vi "ELVIS III v1.0 Unreserve DI Block.vi"(7 "Allow multiple opens?":bool, 8 "error in (no error)":errorcluster, 10 "DI (N Samples) Channel List":T2, 11 "Generic FPGA Reference":T1) -> (0 "error out":errorcluster)   [LabVIEW 2021]
uses:
  <vilib>/myRIO/Common/Instrument Driver Framework/myRIO v1.0/DI Block/typedefs/DI Block Channels List.ctl
  <vilib>/myRIO/Common/Instrument Driver Framework/myRIO v1.0/DI Block/typedefs/DI Block Channels Enum.ctl
  <vilib>/myRIO/Common/Instrument Driver Framework/Utilities/typedefs/Generic FPGA Reference.ctl
  <vilib>/myRIO/Common/Instrument Driver Framework/ELVIS III v1.0/Resource Manager/vis/ELVIS III v1.0 Create Configuration List.vi
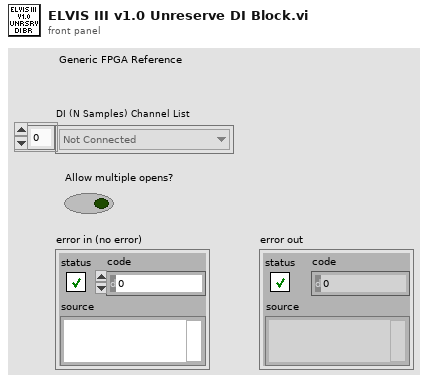
[diagram p1: front panel]
types:
  T1 = typedef "Generic FPGA Reference.ctl" = refnum<k20>
  T2 = typedef "DI Block Channels List.ctl" = T3[]
  T3 = typedef "DI Block Channels Enum.ctl" = enum16{"Not Connected", "A/DI0 (N Samples)", "A/DI1 (N Samples)", "A/DI2 (N Samples)", "A/DI3 (N Samples)", "A/DI4 (N Samples)", "A/DI5 (N Samples)", "A/DI6 (N Samples)", "A/DI7 (N Samples)", "A/DI8 (N Samples)", "A/DI9 (N Samples)", "A/DI10 (N Samples)", "A/DI11 (N Samples)", "A/DI12 (N Samples)", "A/DI13 (N Samples)", "A/DI14 (N Samples)", "A/DI15 (N Samples)", "A/DI16 (N Samples)", "A/DI17 (N Samples)", "A/DI18 (N Samples)", "A/DI19 (N Samples)", "B/DI0 (N Samples)", "B/DI1 (N Samples)", "B/DI2 (N Samples)", "B/DI3 (N Samples)", "B/DI4 (N Samples)", "B/DI5 (N Samples)", "B/DI6 (N Samples)", "B/DI7 (N Samples)", "B/DI8 (N Samples)", "B/DI9 (N Samples)", "B/DI10 (N Samples)", "B/DI11 (N Samples)", "B/DI12 (N Samples)", "B/DI13 (N Samples)", "B/DI14 (N Samples)", "B/DI15 (N Samples)", "B/DI16 (N Samples)", "B/DI17 (N Samples)", "B/DI18 (N Samples)", "B/DI19 (N Samples)"}
  T4 = typedef "ELVIS III v1.0 Channel Reservation List.ctl" = T5[]
  T5 = typedef "ELVIS III v1.0 Channel Reservation Info.ctl" = cluster{"Channel Name":string, "Connector":T6, "MutexIDs":u32[]}
  T6 = typedef "ELVIS III v1.0 Connector List.ctl" = enum32{"None", "ConnectorA", "ConnectorB"}
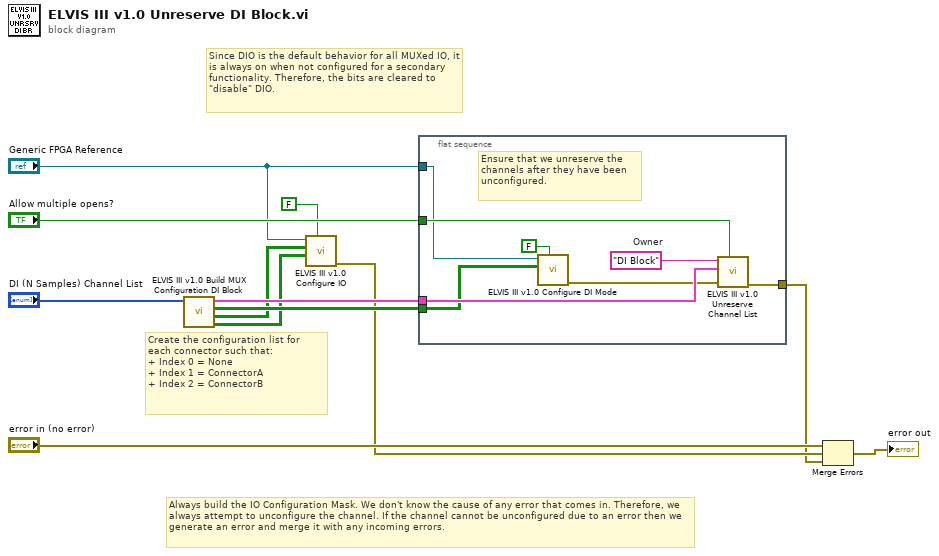
[diagram p0: block diagram]
diagram:
  # "Since DIO is the default behavior for all MUXed IO, it is always on when not configured for a secondary functionality. Therefore, the bits are cleared to \"disable\" DIO."
  # "Always build the IO Configuration Mask. We don't know the cause of any error that comes in. Therefore, we always attempt to unconfigure the channel. If the channel cannot be unconfigured due to an error then we generate an error and merge it with any incoming errors."
  # "Create the configuration list for each connector such that:\n+ Index 0 = None\n+ Index 1 = ConnectorA\n+ Index 2 = ConnectorB"
  n1 = call <vilib>:"ELVIS III v1.0 Build MUX Configuration DI Block.vi"("DI (N Samples) Channel List"="DI (N Samples) Channel List") -> ("Configuration Bitmask Array"=w4:bool[][], "Configration Bitcode Array"=w5:bool[][], "DIO Mode Bitask"=w7:bool[][], "Channel Reservation List"=w8:T4)  [unwired: 7 in]
  n2 = call <vilib>:"ELVIS III v1.0 Configure IO.vi"("Value"=FALSE, "Bitmask Array"=w4, "Bitcode Array"=w5, "myRIO FPGA Ref In"="Generic FPGA Reference") -> ("error out"=w3:errorcluster)  [unwired: 7 in]
  n3 = flat-sequence {
    tunnel: "Allow multiple opens?" -> [w20]
    tunnel: w8 -> [w18]
    tunnel: [w13] -> w2
    tunnel: "Generic FPGA Reference" -> [w16]
    tunnel: w7 -> [w15]
    frame #0 {
      w19 = "DI Block"  # Owner
      # "Ensure that we unreserve the channels after they have been unconfigured."
      n4 = call <vilib>:"ELVIS III v1.0 Configure DI Mode.vi"("Apply Bitmask?"=FALSE ("Set or Reset?"), "Bitmask Array"=w15, "myRIO FPGA Ref In"=w16) -> ("error out"=w14:errorcluster)  [unwired: 8 in]
      n5 = call <vilib>:"ELVIS III v1.0 Unreserve Channel List.vi"("Allow multiple opens?"=w20, "error in (no error)"=w14, "Channel Reservation List"=w18, "Owner"=w19) -> ("error out"=w13:errorcluster)  [unwired: 7 in]
    }
  }
  n6 = Merge Errors("error in (no error)", w3, w2) -> (→"error out":errorcluster)
